vi "ConfigureAcquisition.vi"(8 "error in (no error)":errorcluster, 11 "Keysight44xx in":refnum<class "Keysight44xx.lvclass">) -> (0 "error out":errorcluster, 3 "Keysight44xx out":refnum<class "Keysight44xx.lvclass">)   [LabVIEW 2018, in "SpecAnPlugins.lvlib" / "Keysight44xx.lvclass"]
doc: "This function configures the acquistion attributes of the spectrum analyzer such as\nSweepModeContinuous or NumberofSweeps."
uses:
  Keysight44xx.lvclass
  C:/Users/ico/Documents/Projects/NistPluggableModules/SpecAn/SpecAnPlugins/SpecAnBaseClass/SpecAnBase.lvclass
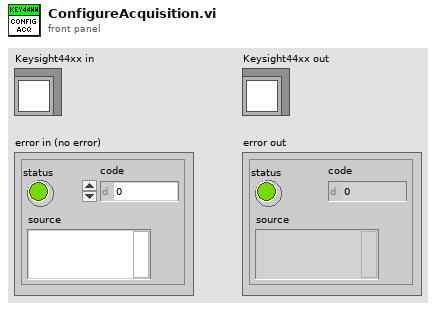
[diagram p1: front panel]
types:
  T1 = typedef "SpecAnPlugins.lvlib/SpecAnBase.lvclass/Acquisition.ctl" = cluster{"Handle":string, "Connected":bool, "Enabled":bool, "SweepModeContinuous":bool, "NumberOfSweeps":i32, "DetectorTypeAuto":bool, "DetectorType":i32, "VerticalScale":i32, "MaximumTime(seconds)":dbl}
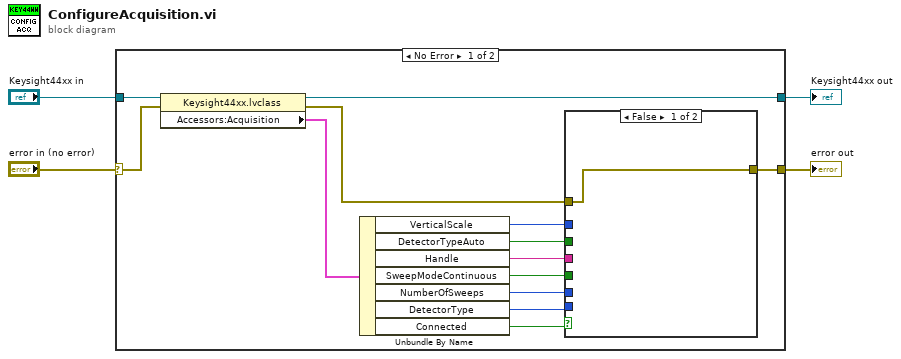
[diagram p0: block diagram]
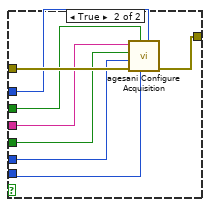
[diagram p2: hidden frame]
diagram:
  n1 = case shown="No Error" "error in (no error)" {
    selector: "error in (no error)" -> [w16 w28]
    tunnel: "Keysight44xx in" -> [w15 w27]
    tunnel: [w17 w28] -> w2
    tunnel: [w13 w27] -> w1
    frame No Error {
      n2 = property class="Keysight44xx.lvclass"(reference=w15, error in=w16) -> (reference out=w13:refnum<class "Keysight44xx.lvclass">, error out=w12:errorcluster, "Accessors:Acquisition"=w14:T1)
      n3 = Unbundle By Name(w14) -> ("VerticalScale"=w9:i32, "DetectorTypeAuto"=w10:bool, "Handle"=w11:string, "SweepModeContinuous"=w8:bool, "NumberOfSweeps"=w7:i32, "DetectorType"=w6:i32, "Connected"=w5:bool)
      n4 = case shown="False" w5 {
        tunnel: [w18 w26] -> w17
        tunnel: w12 -> [w18 w25]
        tunnel: w11 -> [_ w24]
        tunnel: w10 -> [_ w23]
        tunnel: w9 -> [_ w22]
        tunnel: w8 -> [_ w21]
        tunnel: w7 -> [_ w20]
        tunnel: w6 -> [_ w19]
        frame False {
        }
        frame True {
          n5 = call <instrlib>:"agesani Configure Acquisition.vi"("vertical scale (Logarithmic)"=w22, "detector type (Maximum Peak)"=w19, "detector type auto (On)"=w23, "error in (no error)"=w25, "number of sweeps (1)"=w20, "sweep mode continuous (On)"=w21, "instrument handle"=w24) -> ("error out"=w26:errorcluster)  [unwired: 4 out]
        }
      }
    }
    frame Error {
    }
  }
  "error out" <- w2
  "Keysight44xx out" <- w1
